vi "4Pi Dual DM Control.vi"(7 "Calling VI Ref":refnum<vi>) -> ()   [LabVIEW 2016]
uses:
  4Pi Dual DM - Controls/4Pi Dual DM - Mirror Modes.ctl
  4Pi Dual DM - Controls/DM Max Voltages.ctl
  <vilib>/Utility/miscctls.llb/LVPointTypeDef.ctl
  4Pi Dual DM - Controls/4Pi Dual DM - Mirror Order.ctl
  4Pi Dual DM - Controls/4Pi Dual DM - Standard Action.ctl
  <vilib>/Analysis/baseanly.llb/Mean (DBL).vi
  <vilib>/Utility/file.llb/Read Delimited Spreadsheet (DBL).vi
  <vilib>/Utility/file.llb/Write Delimited Spreadsheet (DBL).vi
  <vilib>/Analysis/NI_AALBase.lvlib
panel:
  in  "DM Max Voltages (V)":T1
  in  "Scan Modes":bool
  in  "Astig On/Off":bool
  in  "Load Astig":bool
  in  "Active Mirror":enum32{"Mirror 1", "Mirror 2"}(radio)
  in  "Clear Modes":bool
  in  "Mirror Modes":T2
  in  "Load Modes":bool
  in  "Save Modes":bool
  in  "Load Flat":bool
  in  "Apply Zero":bool
  in  "Load V Map":bool
  in  "Save V Map":bool
  in  "Apply Flat":bool
  in  "Center Bias":bool
  in  "Quit":bool
  out "Pixel Map (-1 to 1)":dbl[][](graph)
  # "Mode"
  # "Amount (nm)"
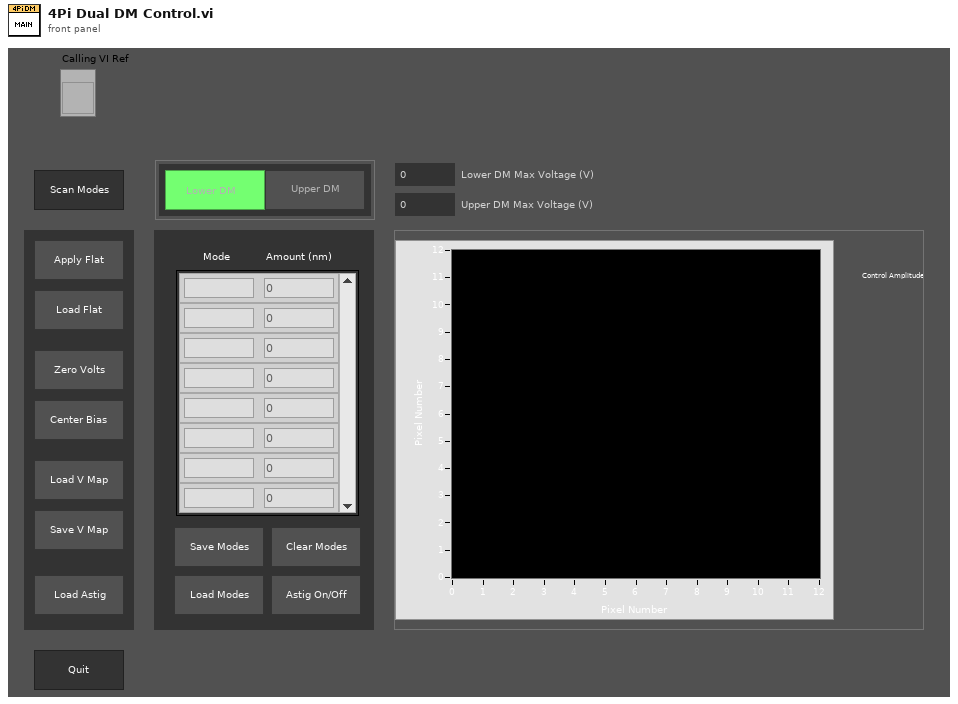
[diagram p1: front panel]
types:
  T1 = typedef "DM Max Voltages.ctl" = cluster{"Lower DM Max Voltage (V)":dbl, "Upper DM Max Voltage (V)":dbl}
  T2 = typedef "4Pi Dual DM - Mirror Modes.ctl" = cluster{"Mode":string, "Amplitude":dbl}[]
  T3 = typedef "4Pi Dual DM - Mirror Order.ctl" = cluster{"Flip Mirror Order":bool}
  T4 = enum16{"Always On", "Always Off", "Off While Running"}
  T5 = typedef "LVPointTypeDef.ctl" = cluster{"Horizontal":i16, "Vertical":i16}
  T6 = typedef "4Pi Dual DM - Standard Action.ctl" = enum16{"Read", "Write"}
  T7 = typedef "LVRectTypeDef.ctl" = cluster{"Left":i16, "Top":i16, "Right":i16, "Bottom":i16}
  T8 = typedef "LVBoundsTypeDef.ctl" = cluster{"Width":u32, "Height":u32}
  T9 = typedef "4Pi Dual DM - Mirror Modes DUAL.ctl" = cluster{"Mode":string, "Amplitude":dbl}[][]
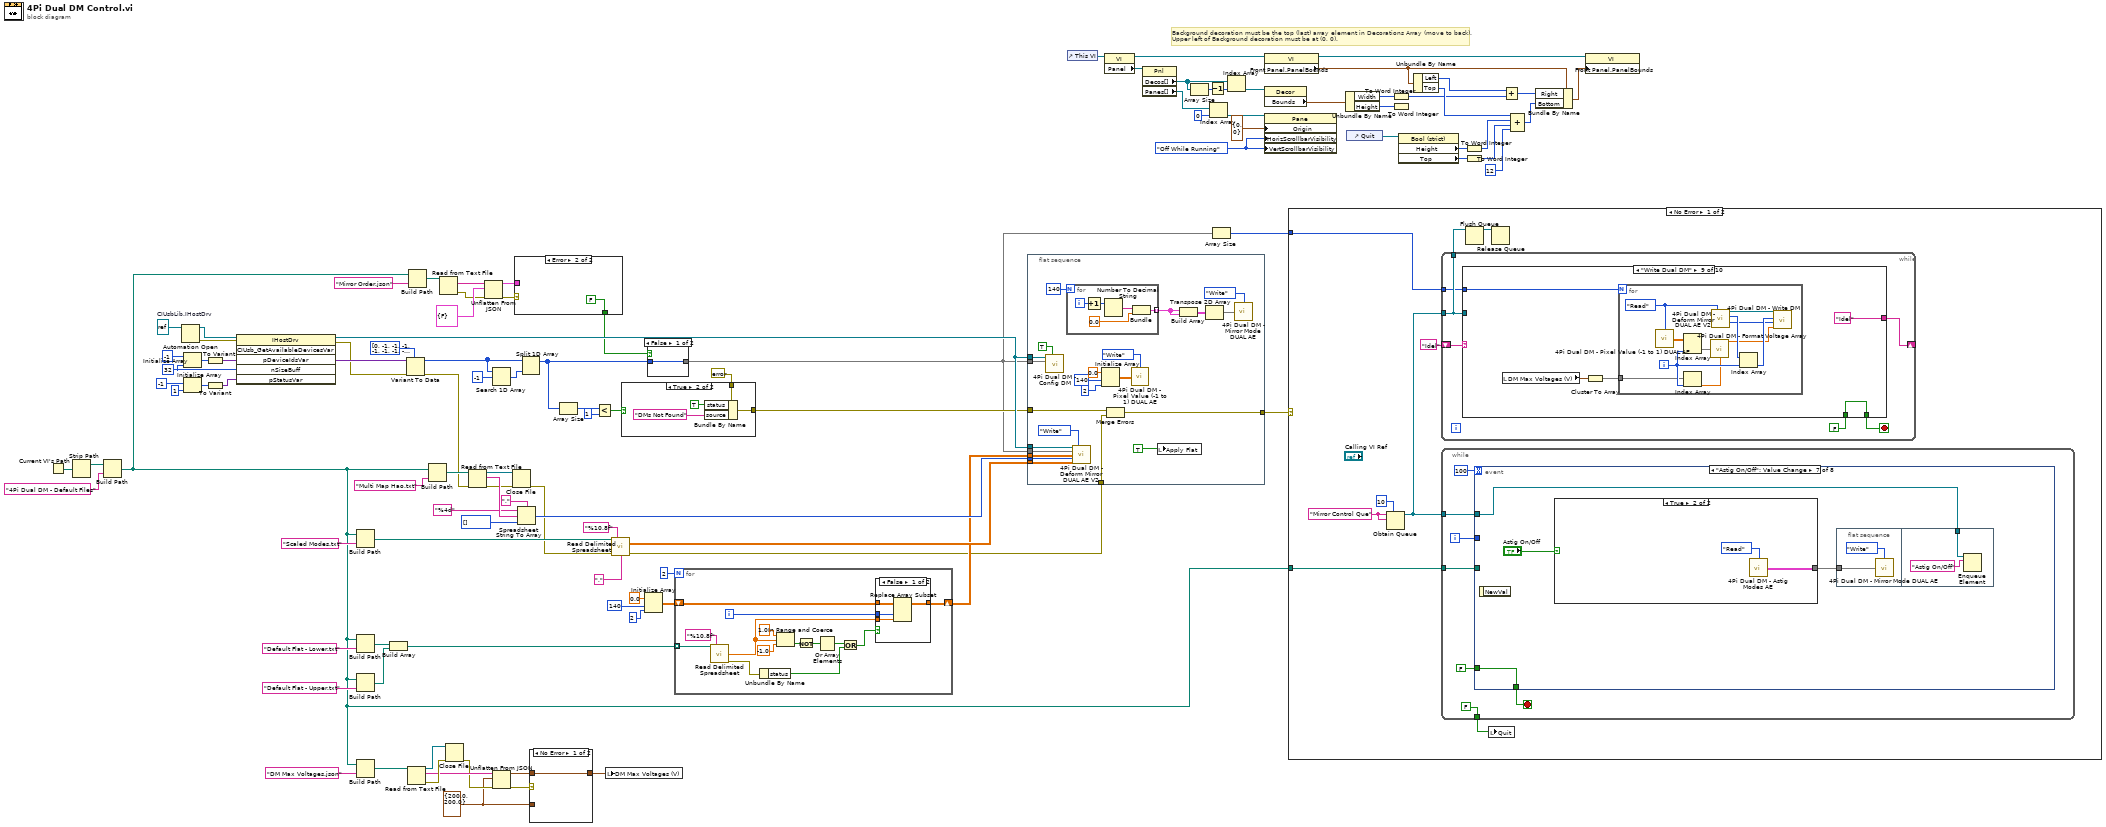
[diagram p0: block diagram]
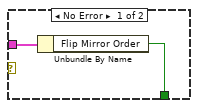
[diagram p2: hidden frame]
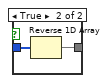
[diagram p4: hidden frame]
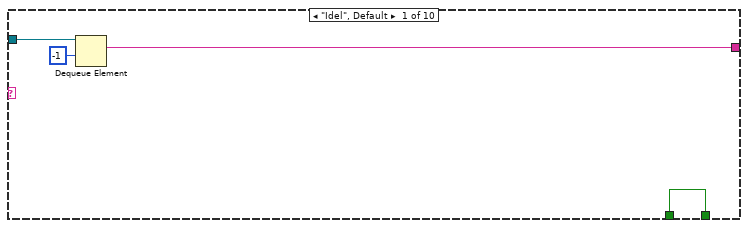
[diagram p5: hidden frame]
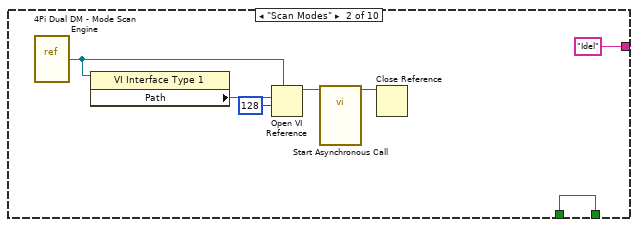
[diagram p6: hidden frame]
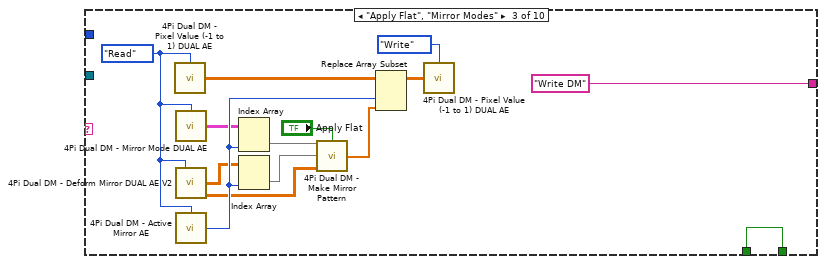
[diagram p7: hidden frame]
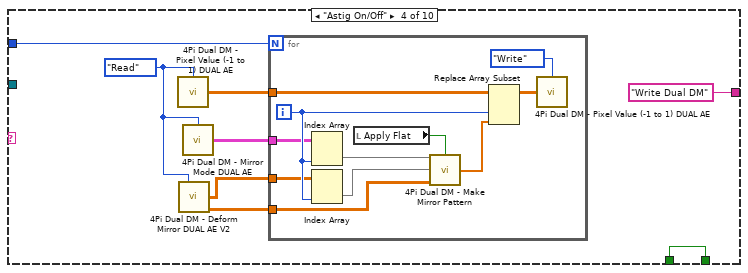
[diagram p8: hidden frame]
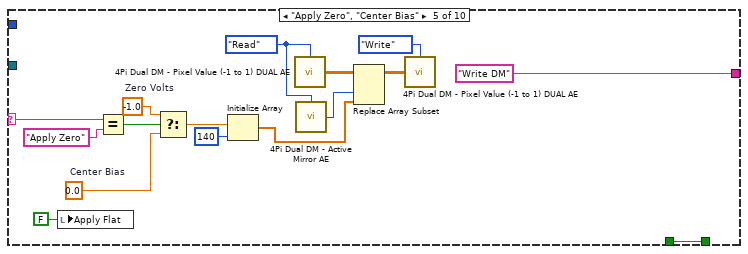
[diagram p9: hidden frame]
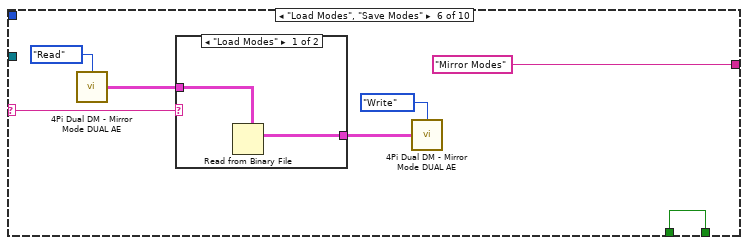
[diagram p10: hidden frame]
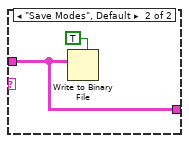
[diagram p11: hidden frame]
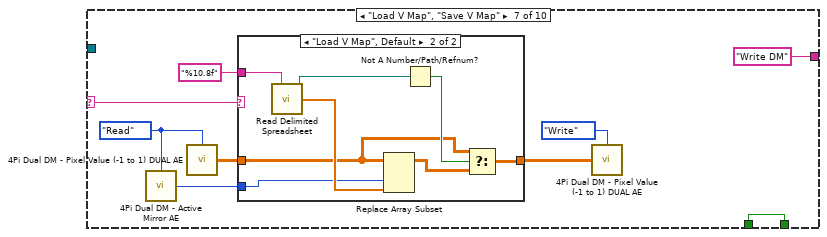
[diagram p12: hidden frame]
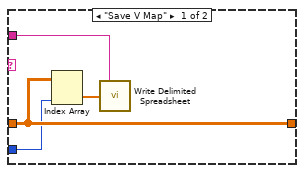
[diagram p13: hidden frame]
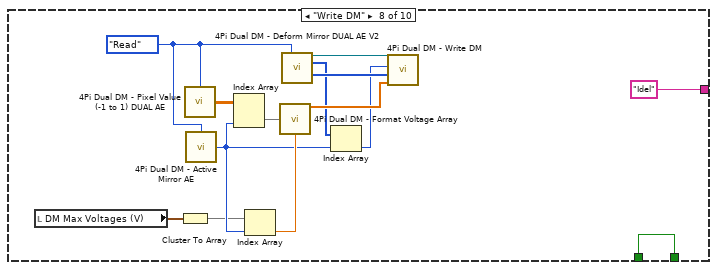
[diagram p14: hidden frame]
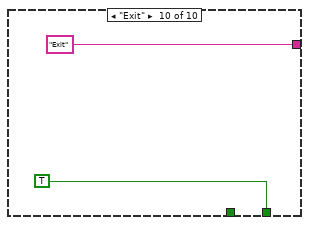
[diagram p15: hidden frame]
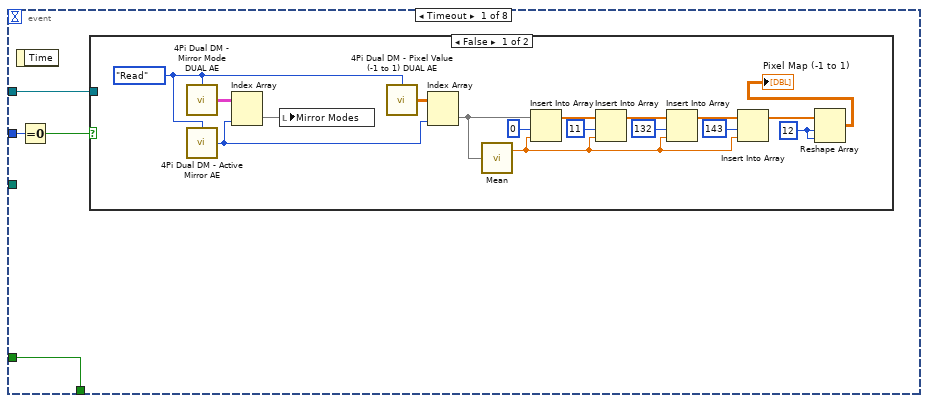
[diagram p16: hidden frame]
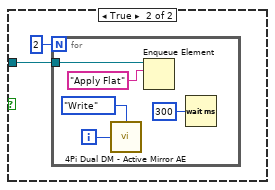
[diagram p17: hidden frame]
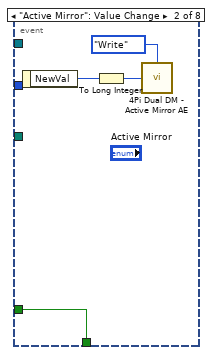
[diagram p18: hidden frame]
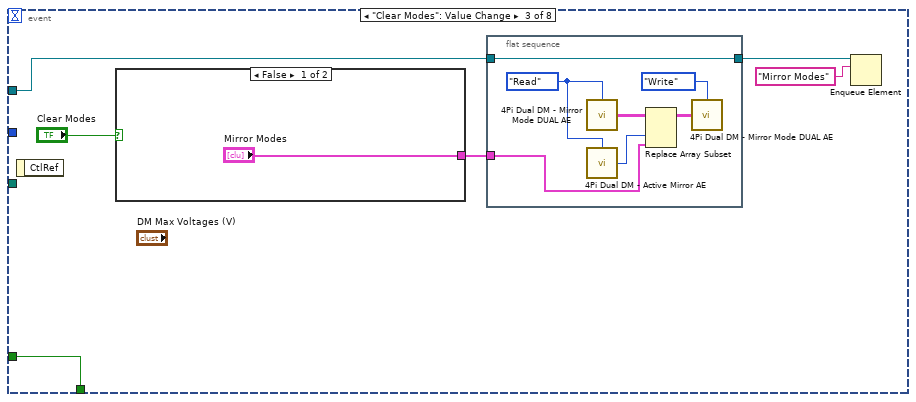
[diagram p19: hidden frame]
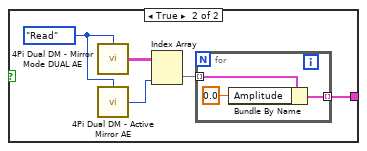
[diagram p20: hidden frame]
diagram:
  w8 = T1 {"Lower DM Max Voltage (V)"=200.0, "Upper DM Max Voltage (V)"=200.0} ("DM Max Voltages (V)")
  w72 = 32 ("dimension size")
  w63 = refnum<k7> refnum  # CIUsbLib.IHostDrv
  w89 = T4."Off While Running" ("Vertical Scrollbar Visibility")
  # "Background decoration must be the top (last) array element in Decorations Array (move to back).\nUpper left of Background decoration must be at (0, 0)."
  n1 = Current VI's Path() -> (path=w47:path)
  n2 = Strip Path(path=w47) -> (stripped path=w48:path)  [unwired: 1 out]
  n3 = Build Path(base path=w48, name or relative path="4Pi Dual DM - Default Files") -> (appended path=w3:path)
  n4 = Automation Open(Automation Refnum=w63) -> (Automation Refnum=w68:refnum<k7>, error out=w69:errorcluster)  [unwired: 1 in, 2 out]
  n5 = Initialize Array(-1 ("element"), w72) -> (w65:i32[])
  n6 = Initialize Array(-1 ("element"), 1 ("dimension size")) -> (w64:i32[])
  n7 = To Variant(anything=w65) -> (Variant=w66:variant)
  n8 = To Variant(anything=w64) -> (Variant=w71:variant)
  n9 = invoke class="IHostDrv" method="CIUsb_GetAvailableDevicesVar"(reference=w68, error in=w69, "pDeviceIdsVar"=w66, "nSizeBuff"=w72, "pStatusVar"=w71) -> (reference out=w25:refnum<k7>, error out=w43:errorcluster, "pDeviceIdsVar"=w77:variant)  [unwired: 1 in, 3 out]
  n10 = Build Path(base path=w3, name or relative path="Scaled Modes.txt") -> (appended path=w54:path)
  n11 = Build Path(base path=w3, name or relative path="Default Flat - Lower.txt") -> (appended path=w35:path)
  n12 = Build Path(base path=w3, name or relative path="Default Flat - Upper.txt") -> (appended path=w34:path)
  n13 = Build Path(base path=w3, name or relative path="DM Max Voltages.json") -> (appended path=w14:path)
  n14 = Build Array(w35, w34) -> (w33:path[])
  n15 = Variant To Data(error in=w43, type=i32[] [0, -1, -1, -1, -1, -1, -1, -1, -1, -1, -1, -1, -1, -1, -1, -1, -1, -1, -1, -1, -1, -1, -1, -1, -1, -1, -1, -1, -1, -1, -1, -1] ("pDeviceIDs"), Variant=w77) -> (data=w75:i32[], error out=w31:errorcluster)
  n16 = Read from Text File(file (use dialog)=w14) -> (refnum out=w13:refnum<file>, text=w11:string, error out=w12:errorcluster)  [unwired: 3 in, 1 out]
  n17 = Build Path(base path=w3, name or relative path="Mirror Order.json") -> (appended path=w21:path)
  n18 = Build Path(base path=w3, name or relative path="Multi Map Hao.txt") -> (appended path=w56:path)
  n19 = Read from Text File(file (use dialog)=w21) -> (text=w20:string, error out=w16:errorcluster)  [unwired: 3 in, 2 out]
  n20 = Close File(refnum=w13, error in=w12) -> (error out=w10:errorcluster)  [unwired: 1 out]
  n21 = Read from Text File(file (use dialog)=w56, error in=w31) -> (refnum out=w58:refnum<file>, text=w62:string, error out=w57:errorcluster)  [unwired: 3 out]
  n22 = Unflatten From JSON(JSON string=w20, type and defaults=T3 {"Flip Mirror Order"=FALSE} ("Mirror Order"), error in (no error)=w16) -> (value=w18:T3, error out=w4:errorcluster)  [unwired: 4 in]
  n23 = Search 1D Array(1D array=w75, element=-1) -> (index of element=w74:i32)  [unwired: 1 in]
  n24 = Unflatten From JSON(JSON string=w11, type and defaults=w8, error in (no error)=w10) -> (value=w7:T1, error out=w9:errorcluster)  [unwired: 4 in]
  n25 = Close File(refnum=w58, error in=w57) -> (error out=w30:errorcluster)  [unwired: 1 out]
  n26 = case shown="Error" w4 {
    tunnel: w18 -> [w108 _]
    tunnel: [w107 FALSE ("Flip Mirror Order")] -> w17
    frame No Error {
      n27 = Unbundle By Name(w108) -> ("Flip Mirror Order"=w107:bool)
    }
    frame Error {
    }
  }
  n28 = Spreadsheet String To Array(delimiter (Tab)=",", format string="%4d", spreadsheet string=w62, array type (2D Dbl)=i32[] []) -> (array=w50:i32[])
  n29 = Split 1D Array(array=w75, index=w74) -> (first subarray=w49:i32[])  [unwired: 1 out]
  n30 = case shown="No Error" w9 {
    tunnel: w8 -> [_ w111]
    tunnel: w7 -> [w110 _]
    tunnel: [w110 w111] -> w6
    frame No Error {
    }
    frame Error {
    }
  }
  n31 = Array Size(array=w49) -> (size(s)=w29:i32)
  n32 = Less?(x=w29, y=1) -> (x < y?=w27:bool)
  n33 = local write "DM Max Voltages (V)"(w6) -> ()
  n34 = call-poly <vilib>:"Read Delimited Spreadsheet.vi"("file path (dialog if empty)"=w54, "format (%.3f)"="%10.8f", "error in (no error)"=w30, "delimiter (\\t)"="," ("delimiter (\\t)")) -> ("all rows"=w52:dbl[][], "error out"=w23:errorcluster)  [unwired: 6 in, 4 out]
  n35 = case shown="True" w27 {
    tunnel: [w112 w114] -> w5
    tunnel: errorcluster {"status"=FALSE, "code"=0, "source"=""} ("error out") -> [w112 w113]
    frame False {
    }
    frame True {
      n36 = Bundle By Name(cluster=w113, "status"=TRUE, "source"="DMs Not Found" ("message")) -> (w114:errorcluster)
    }
  }
  n37 = Initialize Array(0.0 ("element"), 140 ("dimension size"), 2 ("dimension size")) -> (w38:dbl[][])
  n38 = case shown="False" w17 {
    tunnel: w49 -> [w117 w119]
    tunnel: [w117 w118] -> w2
    frame False {
    }
    frame True {
      n39 = Reverse 1D Array(array=w119) -> (reversed array=w118:i32[])
    }
  }
  n40 = for {
    N: 2 -> [_]
    shift-right: [w130] -> w32
    shift-left: w38 -> [w133]
    tunnel: w33 -> [w124] mode=indexing
    i -> [w132]
    n41 = call-poly <vilib>:"Read Delimited Spreadsheet.vi"("file path (dialog if empty)"=w124, "format (%.3f)"="%10.8f") -> ("first row"=w125:dbl[], "error out"=w123:errorcluster)  [unwired: 8 in, 4 out]
    n42 = Unbundle By Name(w123) -> ("status"=w121:bool)
    n43 = In Range and Coerce(upper limit=1.0, x=w125, lower limit=-1.0) -> (In Range?=w127:bool[])  [unwired: 1 out]
    n44 = Not(x=w127) -> (.not. x?=w128:bool[])
    n45 = Or Array Elements(Boolean array=w128) -> (logical OR=w122:bool)
    n46 = Or(x=w122, y=w121) -> (x .or. y?=w120:bool)
    n47 = case shown="False" w120 {
      tunnel: w133 -> [w137 w138]
      tunnel: w132 -> [w136 _]
      tunnel: [w135 w138] -> w130
      tunnel: w125 -> [w134 _]
      frame False {
        n48 = Replace Array Subset(array=w137, new element=w134, index (col)=w136) -> (w135:dbl[][])  [unwired: 1 in]
      }
      frame True {
      }
    }
  }
  n49 = flat-sequence {
    tunnel: w25 -> [w160]
    tunnel: w52 -> [w158]
    tunnel: w50 -> [w157]
    tunnel: w2 -> [w156]
    tunnel: w32 -> [w155]
    tunnel: w5 -> [w154]
    tunnel: w23 -> [w153]
    tunnel: w25 -> [w152]
    tunnel: [w146] -> w24
    tunnel: w2 -> [w145]
    frame #0 {
      n50 = call "4Pi Dual DM - Config DM.vi"("High Voltage"=TRUE, "Dev IDs"=w156, "Automation Refnum in"=w152) -> ()  [unwired: 7 in, 2 out]
      n51 = for {
        N: 140 -> [_]
        tunnel: [w162] -> w142 mode=indexing
        i -> [w166]
        n52 = Increment(x=w166) -> (x+1=w165:i32)
        n53 = Number To Decimal String(number=w165) -> (decimal integer string=w164:string)  [unwired: 1 in]
        n54 = Bundle(w164, 0.0) -> (w162:cluster{string, dbl})  [unwired: 1 in]
      }
      n55 = call "4Pi Dual DM - Deform Mirror DUAL AE V2.vi"("Refnum In"=w160, "Action"=4Pi_Dual_DM_-_Standard_Action."Write", "IDs In"=w145, "Flat Files In"=w155, "Multi Map Data In"=w157, "Mode Matrix"=w158) -> ()  [unwired: 5 in, 5 out]
      n56 = Initialize Array(0.0 ("element"), 140 ("dimension size"), 2 ("dimension size")) -> (w150:dbl[][])
      n57 = Merge Errors(w154, w153) -> (w146:errorcluster)
      n58 = call "4Pi Dual DM - Pixel Value (-1 to 1) DUAL AE.vi"("Action"=4Pi_Dual_DM_-_Standard_Action."Write", "Pixel Value (-1 to 1)"=w150) -> ()  [unwired: 13 in, 1 out]
      n59 = local write "Apply Flat"(TRUE ("Apply Flat")) -> ()
      n60 = Build Array(w142, w142) -> (w143:cluster{string, dbl}[][])
      n61 = Transpose 2D Array(2D array=w143) -> (transposed array=w144:cluster{string, dbl}[][])
      n62 = call "4Pi Dual DM - Mirror Mode DUAL AE.vi"("Action"=4Pi_Dual_DM_-_Standard_Action."Write", "Mirror Modes In"=w144) -> ()  [unwired: 13 in, 1 out]
    }
  }
  n63 = control-ref of="This VI"() -> (w81:refnum<vi>)
  n64 = property class="VI"(reference=w81) -> (reference out=w90:refnum<vi>, "Panel"=w82:refnum<vi>)  [unwired: 1 in, 1 out]
  n65 = property class="Pnl"(reference=w82) -> ("Decos[]"=w80:refnum<vi>[], "Panes[]"=w86:refnum<vi>[])  [unwired: 1 in, 2 out]
  n66 = Array Size(array=w80) -> (size(s)=w78:i32)
  n67 = Decrement(x=w78) -> (x-1=w79:i32)
  n68 = Index Array(array=w86, index=0) -> (element=w85:refnum<vi>)
  n69 = Array Size(array=w2) -> (size(s)=w1:i32)
  n70 = Index Array(array=w80, index=w79) -> (element=w88:refnum<vi>)
  n71 = property class="VI"(reference=w90) -> (reference out=w92:refnum<vi>, "Front Panel.PanelBounds"=w93:T7)  [unwired: 1 in, 1 out]
  n72 = property class="Decor"(reference=w88) -> ("Bounds"=w91:T8)  [unwired: 1 in, 2 out]
  n73 = property class="Pane"(reference=w85, "Origin"=T5 {"Horizontal"=0, "Vertical"=0}, "HorizScrollbarVisibility"=w89, "VertScrollbarVisibility"=w89) -> ()  [unwired: 1 in, 2 out]
  n74 = case shown="No Error" w24 {
    tunnel: w3 -> [w168 _]
    tunnel: w1 -> [w167 _]
    frame No Error {
      w175 = "Mirror Control Que" ("name (unnamed)")
      n75 = Obtain Queue(max queue size (-1, unlimited)=10, name (unnamed)=w175, element data type=w175) -> (queue out=w170:refnum<queue>)  [unwired: 2 in, 2 out]
      n76 = while {
        tunnel: w170 -> [w177]
        shift-right: [w181] -> _
        shift-left: "Idel" ("name (unnamed)") -> [w180]
        tunnel: [w177] -> w173
        tunnel: w167 -> [w176]
        stop <- w179 stop-if-true
        n77 = case shown="\"Write Dual DM\"" w180 {
          selector: w180 -> [_ _ _ _ w237 w244 w260 _ _ _]
          tunnel: w177 -> [w185 _ _ _ _ _ _ _ _ _]
          tunnel: [w183 "Idel" ("name (unnamed)") "Write DM" ("name (unnamed)") "Write Dual DM" ("name (unnamed)") "Write DM" ("name (unnamed)") "Mirror Modes" ("name (unnamed)") "Write DM" ("name (unnamed)") "Idel" ("name (unnamed)") "Idel" ("name (unnamed)") "Exit" ("name (unnamed)")] -> w181
          tunnel: [w182 w192 w205 w213 w241 w248 w261 w287 w292 TRUE] -> w179
          tunnel: FALSE -> [w182 w192 w205 w213 w241 w248 w261 w287 w292 _]
          tunnel: w176 -> [_ _ _ w207 _ _ _ _ w288 _]
          frame "Idel", Default {
            n78 = Dequeue Element(queue=w185, timeout in ms (-1)=-1) -> (element=w183:string)  [unwired: 1 in, 3 out]
          }
          frame "Scan Modes" {
            n79 = vi-ref "4Pi Dual DM - Mode Scan Engine.vi"() -> (w186:refnum<vi>)
            n80 = property class="VI Interface Type 1"(reference=w186) -> ("Path"=w187:path)  [unwired: 1 in, 2 out]
            n81 = Open VI Reference(type specifier VI Refnum (for type only)=w186, vi path=w187, options=128) -> (vi reference=w189:refnum<vi>)  [unwired: 3 in, 1 out]
            n82 = call-by-ref "Start Asynchronous Call"(reference=w189) -> (reference out=w190:refnum<vi>)  [unwired: 17 in, 1 out]
            n83 = Close Reference(reference=w190) -> ()  [unwired: 1 in, 1 out]
          }
          frame "Apply Flat", "Mirror Modes" {
            w200 = 4Pi_Dual_DM_-_Standard_Action."Read" ("Action")
            n84 = call "4Pi Dual DM - Pixel Value (-1 to 1) DUAL AE.vi"("Action"=w200) -> ("Pixel Value (-1 to 1) Out"=w201:dbl[][])  [unwired: 14 in]
            n85 = call "4Pi Dual DM - Mirror Mode DUAL AE.vi"("Action"=w200) -> ("Mirror Modes Out"=w197:T9)  [unwired: 14 in]
            n86 = call "4Pi Dual DM - Deform Mirror DUAL AE V2.vi"("Action"=w200) -> ("Flat Files Out"=w195:dbl[][], "Mode Matrix Out"=w194:dbl[][])  [unwired: 10 in, 3 out]
            n87 = call "4Pi Dual DM - Active Mirror AE.vi"("Action"=w200) -> ("Active Mirror"=w203:i32)  [unwired: 14 in]
            n88 = Index Array(array=w197, index (col)=w203) -> (element=w198:cluster{"Mode":string, "Amplitude":dbl}[])  [unwired: 1 in]
            n89 = Index Array(array=w195, index (col)=w203) -> (element=w196:dbl[])  [unwired: 1 in]
            n90 = call "4Pi Dual DM - Make Mirror Pattern.vi"("Mirror Modes In"=w198, "Flat On?"="Apply Flat", "Flat File In"=w196, "Mirror Modes Array"=w194) -> ("Pixel Value U (-1 to 1)"=w202:dbl[])  [unwired: 11 in]
            n91 = Replace Array Subset(array=w201, new element=w202, index (col)=w203) -> (w204:dbl[][])  [unwired: 1 in]
            n92 = call "4Pi Dual DM - Pixel Value (-1 to 1) DUAL AE.vi"("Action"=4Pi_Dual_DM_-_Standard_Action."Write", "Pixel Value (-1 to 1)"=w204) -> ()  [unwired: 13 in, 1 out]
          }
          frame "Astig On/Off" {
            w212 = 4Pi_Dual_DM_-_Standard_Action."Read" ("Action")
            n93 = call "4Pi Dual DM - Pixel Value (-1 to 1) DUAL AE.vi"("Action"=w212) -> ("Pixel Value (-1 to 1) Out"=w211:dbl[][])  [unwired: 14 in]
            n94 = call "4Pi Dual DM - Deform Mirror DUAL AE V2.vi"("Action"=w212) -> ("Flat Files Out"=w209:dbl[][], "Mode Matrix Out"=w208:dbl[][])  [unwired: 10 in, 3 out]
            n95 = call "4Pi Dual DM - Mirror Mode DUAL AE.vi"("Action"=w212) -> ("Mirror Modes Out"=w210:T9)  [unwired: 14 in]
            n96 = for {
              N: w207 -> [_]
              tunnel: w211 -> [w218]
              tunnel: w210 -> [w217]
              tunnel: w209 -> [w216]
              tunnel: w208 -> [w215]
              i -> [w219]
              n97 = Index Array(array=w217, index (col)=w219) -> (element=w224:cluster{"Mode":string, "Amplitude":dbl}[])  [unwired: 1 in]
              n98 = Index Array(array=w216, index (col)=w219) -> (element=w225:dbl[])  [unwired: 1 in]
              n99 = local read "Apply Flat"() -> (w220:bool)
              n100 = call "4Pi Dual DM - Make Mirror Pattern.vi"("Mirror Modes In"=w224, "Flat On?"=w220, "Flat File In"=w225, "Mirror Modes Array"=w215) -> ("Pixel Value U (-1 to 1)"=w222:dbl[])  [unwired: 11 in]
              n101 = Replace Array Subset(array=w218, new element=w222, index (col)=w219) -> (w221:dbl[][])  [unwired: 1 in]
              n102 = call "4Pi Dual DM - Pixel Value (-1 to 1) DUAL AE.vi"("Action"=4Pi_Dual_DM_-_Standard_Action."Write", "Pixel Value (-1 to 1)"=w221) -> ()  [unwired: 13 in, 1 out]
            }
          }
          frame "Apply Zero", "Center Bias" {
            w229 = 4Pi_Dual_DM_-_Standard_Action."Read" ("Action")
            w233 = -1.0  # Zero Volts
            w235 = 0.0  # Center Bias
            n103 = local write "Apply Flat"(FALSE ("Apply Flat")) -> ()
            n104 = Equal?(x=w237, y="Apply Zero") -> (x = y?=w236:bool)
            n105 = Select(t=w233, s=w236, f=w235) -> (s? t:f=w234:dbl)
            n106 = Initialize Array(w234, 140 ("dimension size")) -> (w226:dbl[])
            n107 = call "4Pi Dual DM - Pixel Value (-1 to 1) DUAL AE.vi"("Action"=w229) -> ("Pixel Value (-1 to 1) Out"=w227:dbl[][])  [unwired: 14 in]
            n108 = call "4Pi Dual DM - Active Mirror AE.vi"("Action"=w229) -> ("Active Mirror"=w228:i32)  [unwired: 14 in]
            n109 = Replace Array Subset(array=w227, new element=w226, index (col)=w228) -> (w231:dbl[][])  [unwired: 1 in]
            n110 = call "4Pi Dual DM - Pixel Value (-1 to 1) DUAL AE.vi"("Action"=4Pi_Dual_DM_-_Standard_Action."Write", "Pixel Value (-1 to 1)"=w231) -> ()  [unwired: 13 in, 1 out]
          }
          frame "Load Modes", "Save Modes" {
            n111 = call "4Pi Dual DM - Mirror Mode DUAL AE.vi"("Action"=4Pi_Dual_DM_-_Standard_Action."Read") -> ("Mirror Modes Out"=w243:T9)  [unwired: 14 in]
            n112 = case shown="\"Load Modes\"" w244 {
              tunnel: w243 -> [w250 w251]
              tunnel: [w249 w251] -> w242
              frame "Load Modes" {
                n113 = Read from Binary File(5:w250) -> (2:w249:T9)  [unwired: 5 in, 3 out]
              }
              frame "Save Modes", Default {
                n114 = Write to Binary File(data=w251, 5:TRUE ("prepend array or string size? (T)")) -> ()  [unwired: 4 in, 3 out]
              }
            }
            n115 = call "4Pi Dual DM - Mirror Mode DUAL AE.vi"("Action"=4Pi_Dual_DM_-_Standard_Action."Write", "Mirror Modes In"=w242) -> ()  [unwired: 13 in, 1 out]
          }
          frame "Load V Map", "Save V Map" {
            w254 = 4Pi_Dual_DM_-_Standard_Action."Read" ("Action")
            n116 = call "4Pi Dual DM - Active Mirror AE.vi"("Action"=w254) -> ("Active Mirror"=w253:i32)  [unwired: 14 in]
            n117 = call "4Pi Dual DM - Pixel Value (-1 to 1) DUAL AE.vi"("Action"=w254) -> ("Pixel Value (-1 to 1) Out"=w258:dbl[][])  [unwired: 14 in]
            n118 = case shown="\"Load V Map\", Default" w260 {
              tunnel: w258 -> [w264 w266]
              tunnel: "%10.8f" -> [w265 w273]
              tunnel: [w264 w270] -> w255
              tunnel: w253 -> [w262 w267]
              frame "Save V Map" {
                n119 = Index Array(array=w264, index (col)=w262) -> (element=w263:dbl[])  [unwired: 1 in]
                n120 = call-poly <vilib>:"Write Delimited Spreadsheet.vi"("format (%.3f)"=w265, "1D data"=w263) -> ()  [unwired: 12 in, 2 out]
              }
              frame "Load V Map", Default {
                n121 = call-poly <vilib>:"Read Delimited Spreadsheet.vi"("format (%.3f)"=w273) -> ("new file path (Not A Path if cancelled)"=w272:path, "first row"=w268:dbl[])  [unwired: 9 in, 4 out]
                n122 = Replace Array Subset(array=w266, new element=w268, index (col)=w267) -> (w269:dbl[][])  [unwired: 1 in]
                n123 = Not A Number/Path/Refnum?(number/path/refnum=w272) -> (NaN/Path/Refnum?=w271:bool)
                n124 = Select(t=w266, s=w271, f=w269) -> (s? t:f=w270:dbl[][])
              }
            }
            n125 = call "4Pi Dual DM - Pixel Value (-1 to 1) DUAL AE.vi"("Action"=4Pi_Dual_DM_-_Standard_Action."Write", "Pixel Value (-1 to 1)"=w255) -> ()  [unwired: 13 in, 1 out]
          }
          frame "Write DM" {
            w280 = 4Pi_Dual_DM_-_Standard_Action."Read" ("Action")
            n126 = local read "DM Max Voltages (V)"() -> (w275:T1)
            n127 = Cluster To Array(cluster=w275) -> (array=w274:dbl[])
            n128 = call "4Pi Dual DM - Pixel Value (-1 to 1) DUAL AE.vi"("Action"=w280) -> ("Pixel Value (-1 to 1) Out"=w282:dbl[][])  [unwired: 14 in]
            n129 = call "4Pi Dual DM - Active Mirror AE.vi"("Action"=w280) -> ("Active Mirror"=w276:i32)  [unwired: 14 in]
            n130 = Index Array(array=w282, index (col)=w276) -> (element=w281:dbl[])  [unwired: 1 in]
            n131 = Index Array(array=w274, index=w276) -> (element=w277:dbl)
            n132 = call "4Pi Dual DM - Format Voltage Array.vi"("Pixel Level (-1 to 1)"=w281, "Max DM Voltage"=w277) -> ("Voltage Array (Volts)"=w283:dbl[])  [unwired: 12 in, 1 out]
            n133 = call "4Pi Dual DM - Deform Mirror DUAL AE V2.vi"("Action"=w280) -> ("Refnum Out"=w285:refnum<k7>, "IDs Out"=w279:i32[], "Multi Map Data Out"=w284:i32[])  [unwired: 10 in, 2 out]
            n134 = Index Array(array=w279, index=w276) -> (element=w278:i32)
            n135 = call "4Pi Dual DM - Write DM.vi"("reference in"=w285, "nDevId"=w278, "MultiDM  Mapping"=w284, "Voltage Array in"=w283) -> ()  [unwired: 2 in, 2 out]
          }
          frame "Write Dual DM" {
            n136 = local read "DM Max Voltages (V)"() -> (w290:T1)
            n137 = Cluster To Array(cluster=w290) -> (array=w289:dbl[])
            n138 = for {
              N: w288 -> [_]
              tunnel: w289 -> [w294]
              i -> [w295]
              w301 = 4Pi_Dual_DM_-_Standard_Action."Read" ("Action")
              n139 = call "4Pi Dual DM - Pixel Value (-1 to 1) DUAL AE.vi"("Action"=w301) -> ("Pixel Value (-1 to 1) Out"=w299:dbl[][])  [unwired: 14 in]
              n140 = Index Array(array=w299, index (col)=w295) -> (element=w300:dbl[])  [unwired: 1 in]
              n141 = Index Array(array=w294, index=w295) -> (element=w293:dbl)
              n142 = call "4Pi Dual DM - Format Voltage Array.vi"("Pixel Level (-1 to 1)"=w300, "Max DM Voltage"=w293) -> ("Voltage Array (Volts)"=w298:dbl[])  [unwired: 12 in, 1 out]
              n143 = call "4Pi Dual DM - Deform Mirror DUAL AE V2.vi"("Action"=w301) -> ("Refnum Out"=w296:refnum<k7>, "IDs Out"=w302:i32[], "Multi Map Data Out"=w297:i32[])  [unwired: 10 in, 2 out]
              n144 = Index Array(array=w302, index=w295) -> (element=w303:i32)
              n145 = call "4Pi Dual DM - Write DM.vi"("reference in"=w296, "nDevId"=w303, "MultiDM  Mapping"=w297, "Voltage Array in"=w298) -> ()  [unwired: 2 in, 2 out]
            }
          }
          frame "Exit" {
          }
        }
      }
      n146 = while {
        tunnel: w170 -> [w308]
        tunnel: [FALSE] -> w169
        tunnel: w168 -> [w306]
        i -> [w309]
        stop <- w312 stop-if-true
        n147 = event shown="[6] \"Astig On/Off\": Value Change" {
          selector: _ -> [_ _ _ _ _ _ _ _]
          dyn-events: _ -> [_ _ _ _ _ _ _ _]
          timeout: 100 -> [_ _ _ _ _ _ _ _]
          tunnel: [w316 w344 w350 w370 w375 w399 w408 w437] -> w312
          tunnel: FALSE -> [w316 w344 w350 w370 w375 w399 w408 _]
          tunnel: w309 -> [w315 _ _ _ _ _ _ _]
          tunnel: w308 -> [w313 _ w349 w369 _ _ w405 w435]
          tunnel: w306 -> [_ _ _ _ w374 w397 _ _]
          event Timeout {
            n148 = event-data() -> ()  [unwired: 1 in, 1 out]
            n149 = Equal To 0?(x=w315) -> (x = 0?=w314:bool)
            n150 = case shown="False" w314 {
              tunnel: w313 -> [_ w335]
              frame False {
                w329 = 12 ("dimension size")
                w330 = 4Pi_Dual_DM_-_Standard_Action."Read" ("Action")
                n151 = call "4Pi Dual DM - Mirror Mode DUAL AE.vi"("Action"=w330) -> ("Mirror Modes Out"=w317:T9)  [unwired: 14 in]
                n152 = call "4Pi Dual DM - Active Mirror AE.vi"("Action"=w330) -> ("Active Mirror"=w332:i32)  [unwired: 14 in]
                n153 = Index Array(array=w317, index (col)=w332) -> (element=w318:cluster{"Mode":string, "Amplitude":dbl}[])  [unwired: 1 in]
                n154 = local write "Mirror Modes"(w318) -> ()
                n155 = call "4Pi Dual DM - Pixel Value (-1 to 1) DUAL AE.vi"("Action"=w330) -> ("Pixel Value (-1 to 1) Out"=w331:dbl[][])  [unwired: 14 in]
                n156 = Index Array(array=w331, index (col)=w332) -> (element=w333:dbl[])  [unwired: 1 in]
                n157 = call-poly <vilib>:"Mean.vi"("X"=w333) -> ("mean"=w327:dbl)  [unwired: 1 out]
                n158 = Insert Into Array(array=w333, index=0, new element=w327) -> (w322:dbl[])
                n159 = Insert Into Array(array=w322, index=11, new element=w327) -> (w324:dbl[])
                n160 = Insert Into Array(array=w324, index=132, new element=w327) -> (w326:dbl[])
                n161 = Insert Into Array(array=w326, index=143, new element=w327) -> (w319:dbl[])
                n162 = Reshape Array(w319, w329, w329) -> (→"Pixel Map (-1 to 1)":dbl[][])
              }
              frame True {
                n163 = for {
                  N: 2 -> [_]
                  tunnel: w335 -> [w340]
                  i -> [w336]
                  n164 = call "4Pi Dual DM - Active Mirror AE.vi"("Action"=4Pi_Dual_DM_-_Standard_Action."Write", "Active Mirror In"=w336) -> ()  [unwired: 13 in, 1 out]
                  n165 = Enqueue Element(queue=w340, element="Apply Flat") -> ()  [unwired: 2 in, 3 out]
                  n166 = Wait (ms)(milliseconds to wait=u32 300) -> ()  [unwired: 1 out]
                }
              }
            }
          }
          event "Active Mirror": Value Change {
            n167 = event-data() -> ("NewVal"=w343:enum32{"Mirror 1", "Mirror 2"})  [unwired: 1 in]
            n168 = To Long Integer(number=w343) -> (32bit integer=w342:i32)
            n169 = call "4Pi Dual DM - Active Mirror AE.vi"("Action"=4Pi_Dual_DM_-_Standard_Action."Write", "Active Mirror In"=w342) -> ()  [unwired: 13 in, 1 out]
          }
          event "Clear Modes": Value Change {
            n170 = event-data() -> ()  [unwired: 1 in, 1 out]
            n171 = case shown="False" "Clear Modes" {
              tunnel: ["Mirror Modes" w352] -> w345
              frame False {
              }
              frame True {
                w355 = 4Pi_Dual_DM_-_Standard_Action."Read" ("Action")
                n172 = call "4Pi Dual DM - Mirror Mode DUAL AE.vi"("Action"=w355) -> ("Mirror Modes Out"=w354:T9)  [unwired: 14 in]
                n173 = call "4Pi Dual DM - Active Mirror AE.vi"("Action"=w355) -> ("Active Mirror"=w356:i32)  [unwired: 14 in]
                n174 = Index Array(array=w354, index (col)=w356) -> (element=w353:cluster{"Mode":string, "Amplitude":dbl}[])  [unwired: 1 in]
                n175 = for {
                  tunnel: w353 -> [w359] mode=indexing
                  tunnel: [w357] -> w352 mode=indexing
                  n176 = Bundle By Name(cluster=w359, "Amplitude"=0.0) -> (w357:cluster{"Mode":string, "Amplitude":dbl})
                }
              }
            }
            n177 = flat-sequence {
              tunnel: w345 -> [w360]
              tunnel: w349 -> [w366]
              tunnel: [w366] -> w347
              frame #0 {
                w363 = 4Pi_Dual_DM_-_Standard_Action."Read" ("Action")
                n178 = call "4Pi Dual DM - Mirror Mode DUAL AE.vi"("Action"=w363) -> ("Mirror Modes Out"=w362:T9)  [unwired: 14 in]
                n179 = call "4Pi Dual DM - Active Mirror AE.vi"("Action"=w363) -> ("Active Mirror"=w364:i32)  [unwired: 14 in]
                n180 = Replace Array Subset(array=w362, new element=w360, index (col)=w364) -> (w365:T9)  [unwired: 1 in]
                n181 = call "4Pi Dual DM - Mirror Mode DUAL AE.vi"("Action"=4Pi_Dual_DM_-_Standard_Action."Write", "Mirror Modes In"=w365) -> ()  [unwired: 13 in, 1 out]
              }
            }
            n182 = Enqueue Element(queue=w347, element="Mirror Modes") -> ()  [unwired: 2 in, 3 out]
          }
          event "Apply Flat", "Center Bias", "Apply Zero", "Save V Map", "Save Modes", "Load Modes", "Load V Map", "Scan Modes": Value Change {
            n183 = event-data() -> ("CtlRef"=w368:refnum<vi>)  [unwired: 1 in]
            n184 = property class="Bool"(reference=w368) -> ("Label.Text"=w367:string)  [unwired: 1 in, 2 out]
            n185 = Enqueue Element(queue=w369, element=w367) -> ()  [unwired: 2 in, 3 out]
          }
          event "Load Flat": Value Change {
            n186 = event-data() -> ()  [unwired: 1 in, 1 out]
            n187 = call "File Dialog"("start path"=w374, "prompt"="Select Flat File") -> ("selected path"=w371:path, "error out"=w372:errorcluster)  [unwired: 10 in, 2 out]
            n188 = case shown="No Error" w372 {
              tunnel: w371 -> [w376 _]
              frame No Error {
                w383 = 4Pi_Dual_DM_-_Standard_Action."Read" ("Action")
                n189 = call-poly <vilib>:"Read Delimited Spreadsheet.vi"("file path (dialog if empty)"=w376, "format (%.3f)"="%10.8f") -> ("first row"=w392:dbl[])  [unwired: 8 in, 5 out]
                n190 = In Range and Coerce(upper limit=1.0, x=w392, lower limit=-1.0) -> (coerced(x)=w377:dbl[], In Range?=w389:bool[])
                n191 = call "4Pi Dual DM - Deform Mirror DUAL AE V2.vi"("Action"=w383) -> ("Refnum Out"=w378:refnum<k7>, "IDs Out"=w379:i32[], "Flat Files Out"=w384:dbl[][], "Multi Map Data Out"=w380:i32[], "Mode Matrix Out"=w381:dbl[][])  [unwired: 10 in]
                n192 = call "4Pi Dual DM - Active Mirror AE.vi"("Action"=w383) -> ("Active Mirror"=w386:i32)  [unwired: 14 in]
                n193 = Not(x=w389) -> (.not. x?=w388:bool[])
                n194 = Replace Array Subset(array=w384, new element=w377, index (col)=w386) -> (w385:dbl[][])  [unwired: 1 in]
                n195 = Or Array Elements(Boolean array=w388) -> (logical OR=w387:bool)
                n196 = call "4Pi Dual DM - Deform Mirror DUAL AE V2.vi"("Refnum In"=w378, "Action"=4Pi_Dual_DM_-_Standard_Action."Write", "IDs In"=w379, "Flat Files In"=w385, "Multi Map Data In"=w380, "Mode Matrix"=w381) -> ()  [unwired: 5 in, 5 out]
                n197 = case shown="True" w387 {
                  frame False {
                  }
                  frame True {
                    n198 = One Button Dialog(message="Flat File Out of Range [-1, 1]") -> ()  [unwired: 1 in, 1 out]
                  }
                }
              }
              frame Error {
              }
            }
          }
          event "Load Astig": Value Change {
            n199 = event-data() -> ()  [unwired: 1 in, 1 out]
            n200 = call "File Dialog2"("start path"=w397, "prompt"="Select Astigmatism File") -> ("selected path"=w395:path, "error out"=w396:errorcluster)  [unwired: 10 in, 2 out]
            n201 = case shown="No Error" w396 {
              tunnel: w395 -> [w400 _]
              frame No Error {
                n202 = call "4Pi Dual DM - Astig Modes AE.vi"("Action"=4Pi_Dual_DM_-_Standard_Action."Read") -> ("Mirror Modes Out"=w404:T9)  [unwired: 14 in]
                n203 = Read from Binary File(5:w404, 11:w400) -> (2:w401:T9)  [unwired: 4 in, 3 out]
                n204 = call "4Pi Dual DM - Astig Modes AE.vi"("Action"=4Pi_Dual_DM_-_Standard_Action."Write", "Mirror Modes In"=w401) -> ()  [unwired: 13 in, 1 out]
              }
              frame Error {
              }
            }
          }
          event "Astig On/Off": Value Change {
            n205 = event-data() -> ()  [unwired: 1 in, 1 out]
            n206 = case shown="True" "Astig On/Off" {
              tunnel: [w413 w425] -> w406
              frame False {
                n207 = for {
                  N: 2 -> [_]
                  tunnel: [w416] -> w414 mode=indexing
                  i -> [w417]
                  n208 = call "4Pi Dual DM - Mirror Mode DUAL AE.vi"("Action"=4Pi_Dual_DM_-_Standard_Action."Read") -> ("Mirror Modes Out"=w419:T9)  [unwired: 14 in]
                  n209 = Index Array(array=w419, index (col)=w417) -> (element=w420:cluster{"Mode":string, "Amplitude":dbl}[])  [unwired: 1 in]
                  n210 = for {
                    tunnel: w420 -> [w423] mode=indexing
                    tunnel: [w421] -> w416 mode=indexing
                    n211 = Bundle By Name(cluster=w423, "Amplitude"=0.0) -> (w421:cluster{"Mode":string, "Amplitude":dbl})
                  }
                }
                n212 = Transpose 2D Array(2D array=w414) -> (transposed array=w413:cluster{"Mode":string, "Amplitude":dbl}[][])
              }
              frame True {
                n213 = call "4Pi Dual DM - Astig Modes AE.vi"("Action"=4Pi_Dual_DM_-_Standard_Action."Read") -> ("Mirror Modes Out"=w425:T9)  [unwired: 14 in]
              }
            }
            n214 = flat-sequence {
              tunnel: w406 -> [w410]
              tunnel: w405 -> [w411]
              frame #0 {
                n215 = call "4Pi Dual DM - Mirror Mode DUAL AE.vi"("Action"=4Pi_Dual_DM_-_Standard_Action."Write", "Mirror Modes In"=w410) -> ()  [unwired: 13 in, 1 out]
              }
              frame #1 {
                n216 = Enqueue Element(queue=w411, element="Astig On/Off") -> ()  [unwired: 2 in, 3 out]
              }
            }
          }
          event "Quit": Value Change {
            n217 = event-data() -> ("NewVal"=w437:bool)  [unwired: 1 in]
            n218 = for {
              N: 2 -> [_]
              tunnel: w435 -> [w443]
              tunnel: [w438] -> w426
              i -> [w439]
              n219 = call "4Pi Dual DM - Active Mirror AE.vi"("Action"=4Pi_Dual_DM_-_Standard_Action."Write", "Active Mirror In"=w439) -> ()  [unwired: 13 in, 1 out]
              n220 = Enqueue Element(queue=w443, element="Apply Zero") -> (queue out=w438:refnum<queue>)  [unwired: 2 in, 2 out]
              n221 = Wait (ms)(milliseconds to wait=u32 300) -> ()  [unwired: 1 out]
            }
            n222 = Enqueue Element(queue=w426, element="Exit") -> (error out=w430:errorcluster)  [unwired: 2 in, 2 out]
            n223 = call "4Pi Dual DM - Deform Mirror DUAL AE V2.vi"("Action"=4Pi_Dual_DM_-_Standard_Action."Read") -> ("Refnum Out"=w433:refnum<k7>, "IDs Out"=w428:i32[])  [unwired: 10 in, 3 out]
            n224 = call "4Pi Dual DM - Config DM.vi"("High Voltage"=FALSE, "error in (no error)"=w430, "Dev IDs"=w428, "Automation Refnum in"=w433) -> ("error out"=w429:errorcluster, "Automation Refnum out"=w432:refnum<k7>)  [unwired: 6 in]
            n225 = Close Reference(reference=w432, error in (no error)=w429) -> ()  [unwired: 1 out]
          }
        }
      }
      n226 = Flush Queue(queue=w173) -> (queue out=w172:refnum<queue>)  [unwired: 1 in, 2 out]
      n227 = local write "Quit"(w169) -> ()
      n228 = Release Queue(queue=w172) -> ()  [unwired: 2 in, 3 out]
    }
    frame Error {
      n229 = One Button Dialog(message="DMs not found.") -> ()  [unwired: 1 in, 1 out]
    }
  }
  n230 = Unbundle By Name(w91) -> ("Width"=w96:u32, "Height"=w99:u32)
  n231 = control-ref of="Quit"() -> (w83:refnum<vi>)
  n232 = To Word Integer(number=w96) -> (16bit integer=w98:i16)
  n233 = To Word Integer(number=w99) -> ()  [unwired: 1 out]
  n234 = property class="Bool (strict)"(reference=w83) -> ("Height"=w101:u32, "Top"=w102:i32)  [unwired: 1 in, 2 out]
  n235 = Unbundle By Name(w93) -> ("Left"=w95:i16, "Top"=w106:i16)
  n236 = To Word Integer(number=w101) -> (16bit integer=w104:i16)
  n237 = To Word Integer(number=w102) -> (16bit integer=w105:i16)
  n238 = Add(x=w95, y=w98) -> (x+y=w97:i16)
  n239 = Compound Arithmetic op=ADD(w106, w104, w105, i16 12 ("y")) -> (w100:i16)
  n240 = Bundle By Name(cluster=w93, "Right"=w97, "Bottom"=w100) -> (w94:T7)
  n241 = property class="VI"(reference=w92, "Front Panel.PanelBounds"=w94) -> ()  [unwired: 1 in, 2 out]
